vi "plot_counter_data_1.vi"(8 "error in (no error)":errorcluster, 10 "Counter Settings, Tasks and Data":T1, 11 "Cluster":T2) -> (0 "error out":errorcluster)   [LabVIEW 2011]
panel:
  out "Counters Chart 3":u32[][](graph)
  out "counter data":u32[][](array[numeric])
  out "Counters Chart":u32[][](graph)
  out "current counter totals":u32[](array[numeric])
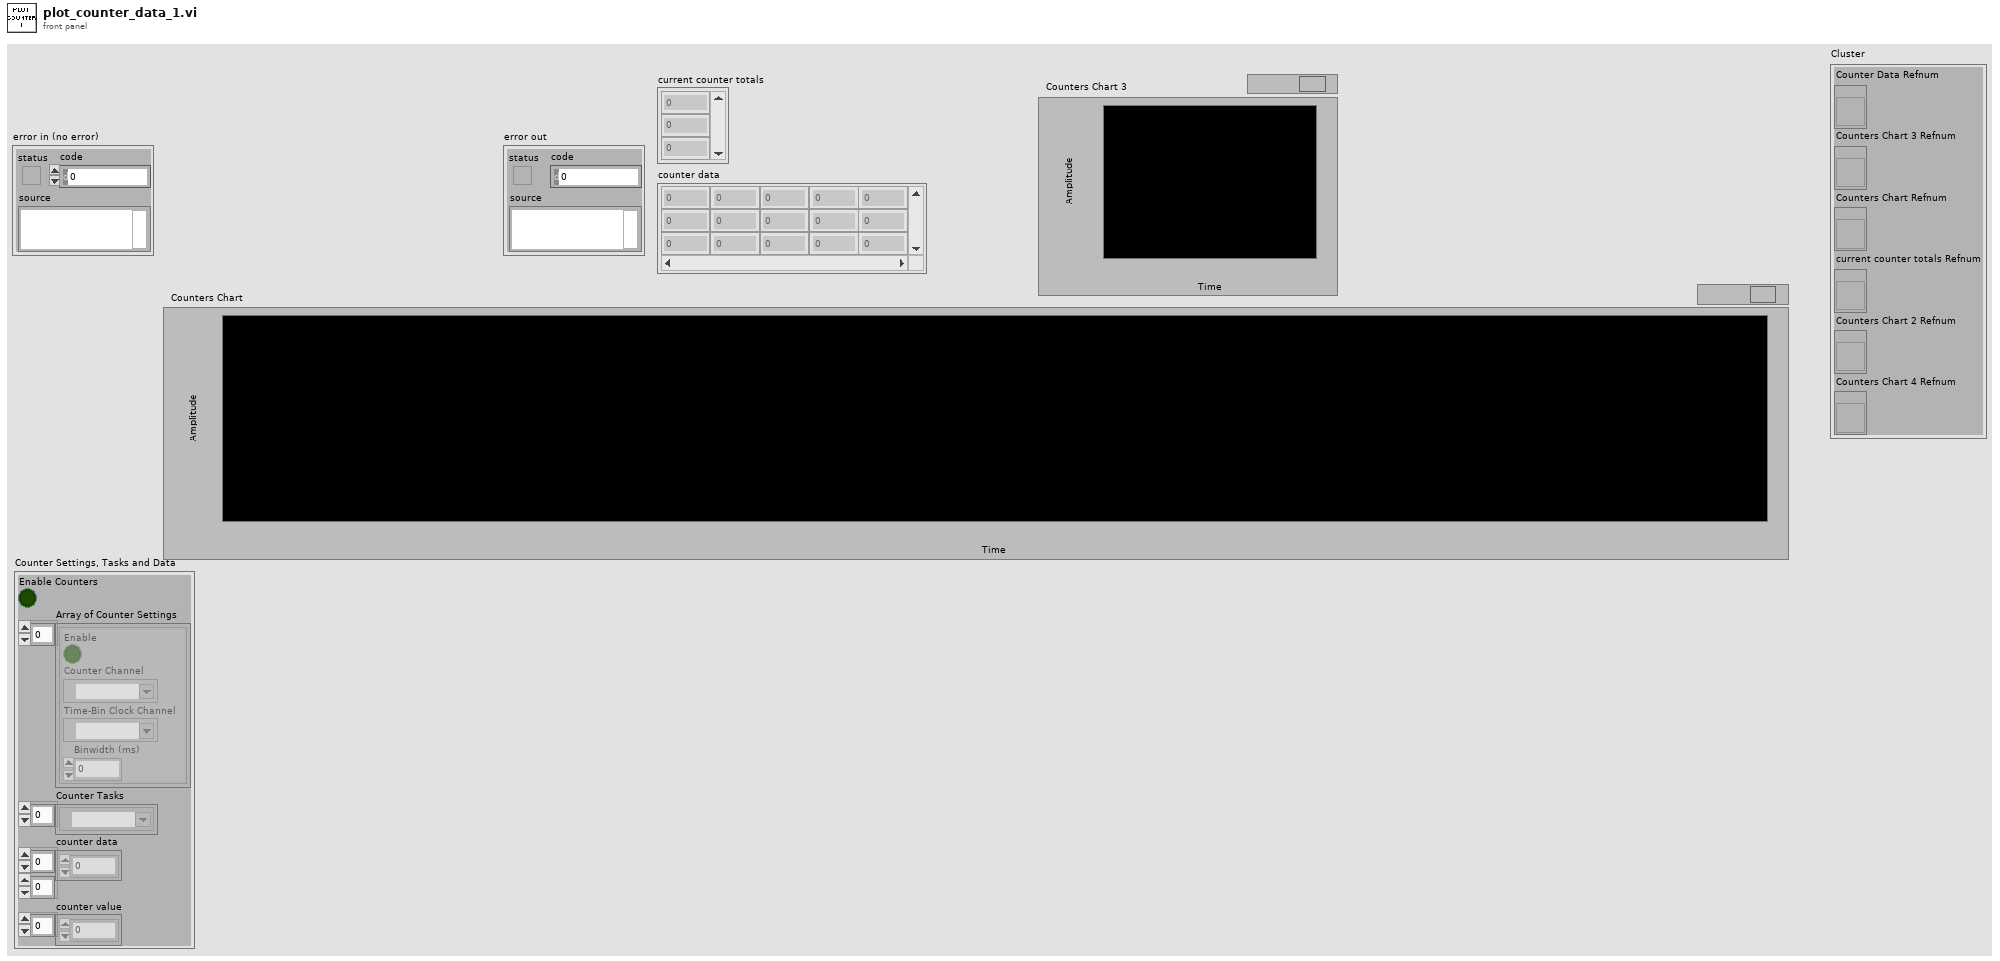
[diagram p1: front panel]
types:
  T1 = cluster{"Enable Counters":bool, "Array of Counter Settings":cluster{"Enable":bool, "Counter Channel":tag, "Time-Bin Clock Channel":tag, "Binwidth (ms)":dbl}[], "Counter Tasks":refnum<k21>[], "counter data":u32[][], "counter value":u32[]}
  T2 = cluster{"Counter Data Refnum":refnum<vi>, "Counters Chart 3 Refnum":refnum<vi>, "Counters Chart Refnum":refnum<vi>, "current counter totals Refnum":refnum<vi>, "Counters Chart 2 Refnum":refnum<vi>, "Counters Chart 4 Refnum":refnum<vi>}
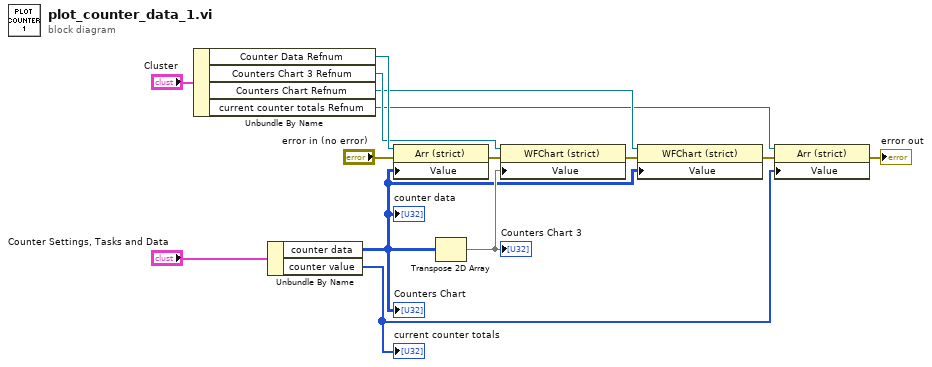
[diagram p0: block diagram]
diagram:
  n1 = Unbundle By Name("Cluster") -> ("Counter Data Refnum"=w13:refnum<vi>, "Counters Chart 3 Refnum"=w12:refnum<vi>, "Counters Chart Refnum"=w11:refnum<vi>, "current counter totals Refnum"=w10:refnum<vi>)
  n2 = Unbundle By Name("Counter Settings, Tasks and Data") -> ("counter data"=w4:u32[][], "counter value"=w3:u32[])
  "current counter totals" <- w3
  "Counters Chart" <- w4
  "counter data" <- w4
  n3 = property class="Arr (strict)"(reference=w13, error in="error in (no error)", "Value"=w4) -> (error out=w9:errorcluster)  [unwired: 1 out]
  n4 = Transpose 2D Array(2D array=w4) -> (transposed array=w5:u32[][])
  "Counters Chart 3" <- w5
  n5 = property class="WFChart (strict)"(reference=w12, error in=w9, "Value"=w5) -> (error out=w8:errorcluster)  [unwired: 1 out]
  n6 = property class="WFChart (strict)"(reference=w11, error in=w8, "Value"=w4) -> (error out=w7:errorcluster)  [unwired: 1 out]
  n7 = property class="Arr (strict)"(reference=w10, error in=w7, "Value"=w3) -> (error out=→"error out":errorcluster)  [unwired: 1 out]
